vi "completeBroadcastSetForceFrame.vi"(0 "FAILC in":refnum<class "FAILC.lvclass">, 5 "FixedFrameBuilder":refnum<class "FixedFrameBuilder.lvclass">, 7 "WaitForTrigger":bool, 9 "TriggerIRQ":bool, 11 "error in (no error)":errorcluster) -> (4 "FAILC out":refnum<class "FAILC.lvclass">, 6 "TxFrame":T1 {"Data" format="%02x"}, 15 "error out":errorcluster)   [LabVIEW 2016, in "RTFAILC.lvlib" / "FAILC.lvclass"]
uses:
  FAILC.lvclass
  Common_RT_Modbus/FixedFrameBuilder/FixedFrameBuilder.lvclass
  Common_RT_Modbus/DataTypes/TxFrame.ctl
  FAILC.lvclass/FAILC.ctl
  Common_RT_Modbus/RTModbus.lvlib
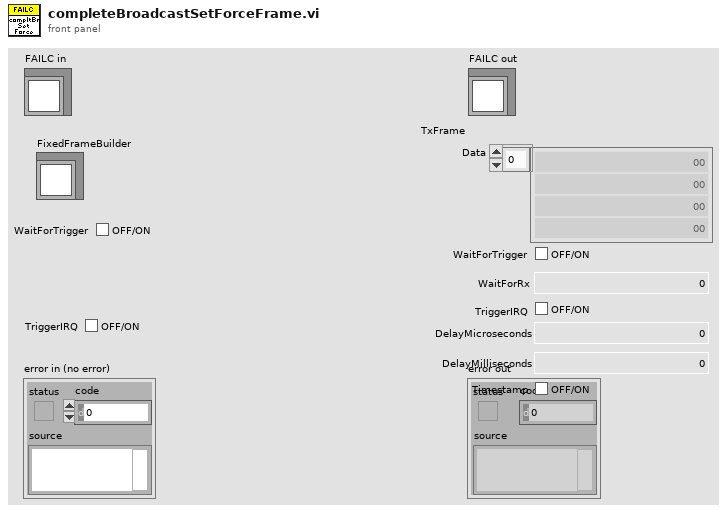
[diagram p1: front panel]
types:
  T1 = typedef "RTModbus.lvlib/TxFrame.ctl" = cluster{"Data":u8[], "WaitForTrigger":bool, "WaitForRx":u16, "TriggerIRQ":bool, "DelayMicroseconds":u16, "DelayMilliseconds":u16, "Timestamp":bool}
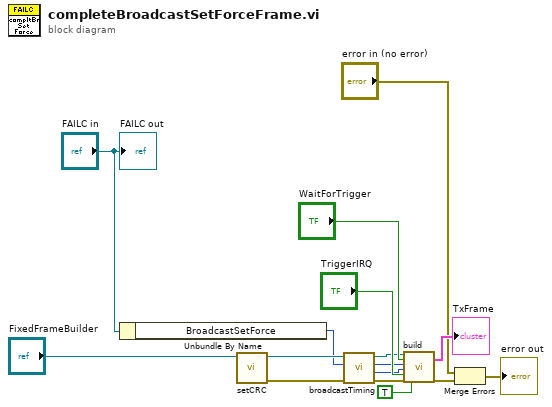
[diagram p0: block diagram]
diagram:
  n1 = Unbundle By Name("FAILC in") -> ("BroadcastSetForce"=w6:u32)
  n2 = call "setCRC.vi"("FixedFrameBuilder in"="FixedFrameBuilder") -> ("error out"=w5:errorcluster, "FixedFrameBuilder out"=w9:refnum<class "FixedFrameBuilder.lvclass">)  [unwired: 9 in]
  n3 = call "broadcastTiming.vi"("error in (no error)"=w5, "Latency in"=w6, "FixedFrameBuilder in"=w9) -> ("error out"=w4:errorcluster, "WaitForRxTimeout"=w2:u16, "Latency out"=w3:u32, "FixedFrameBuilder out"=w8:refnum<class "FixedFrameBuilder.lvclass">)  [unwired: 5 in]
  n4 = call "build.vi"("FixedFrameBuilder in"=w8, "WaitForTrigger"="WaitForTrigger", "Latency"=w3, "WaitForRxTimeout"=w2, "TriggerIRQ"="TriggerIRQ", "error in (no error)"=w4, "Timestamp"=TRUE) -> ("TxFrame"=→"TxFrame":T1, "error out"=w12:errorcluster)  [unwired: 10 in, 1 out]
  n5 = Merge Errors("error in (no error)", w12) -> (→"error out":errorcluster)
  "FAILC out" <- "FAILC in"
